vi "Generic command handler.vi"(8 "error in (no error)":errorcluster, 10 "Message in":refnum<class "GenericMessage.lvclass">, 11 "DAQMH121119OrcaFlash in":refnum<class "DAQOrcaFlash.lvclass">) -> (0 "error out":errorcluster, 2 "value":string, 3 "DAQMH121119OrcaFlash out":refnum<class "DAQOrcaFlash.lvclass">)   [LabVIEW 2012, in "DAQOrcaFlash.lvclass"]
doc: "The generic_command_handler processes the command 'generic'. Commands which are not part of the predefined list of commands fall under the 'generic' command for special activity."
uses:
  DAQOrcaFlash.lvclass
  <vilib>/Distrio/Murmex/GenericMessage/GenericMessage.lvclass
  <vilib>/Distrio/Murmex/Murmex/Murmex.lvclass
  <vilib>/Distrio/Murmex/ResetMessage/ResetMessage.lvclass
  <vilib>/Distrio/Murmex/ProceedMessage/ProceedMessage.lvclass
  DAQOrcaFlash.lvclass/DAQOrcaFlash.ctl
  <vilib>/Distrio/Murmex/Message/Message.lvclass
panel:
  # "This method is called when the GENERIC\ntrigger is sent. \n\nOverride this method when your component needs to\nrespond to this trigger. \n\nCall parent for proper implementation"
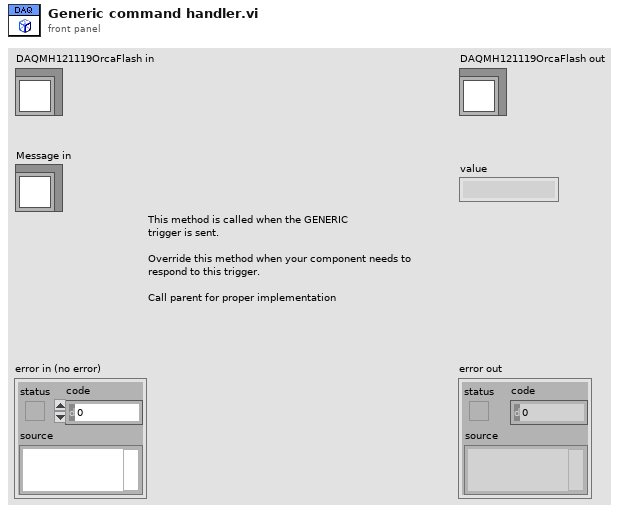
[diagram p1: front panel]
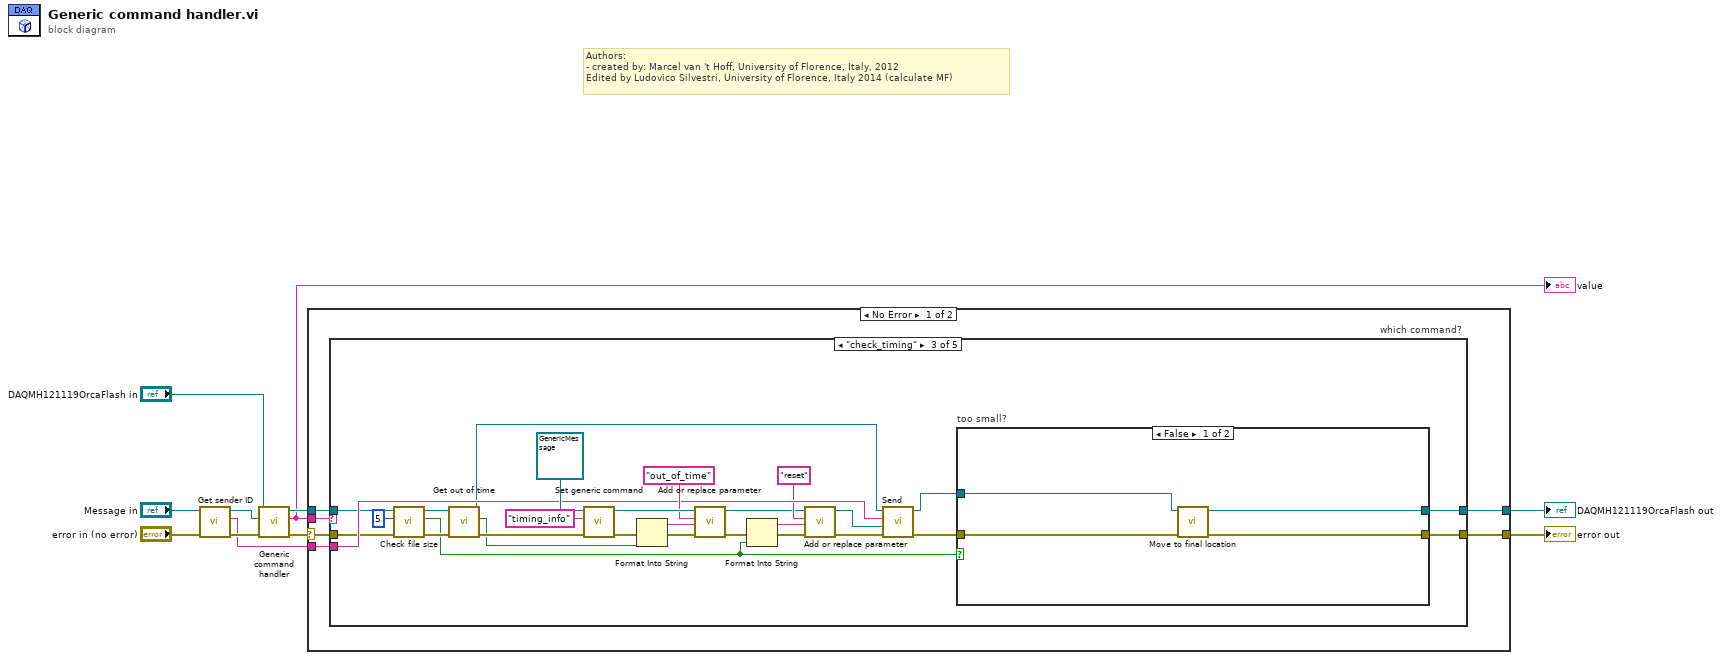
[diagram p0: block diagram]
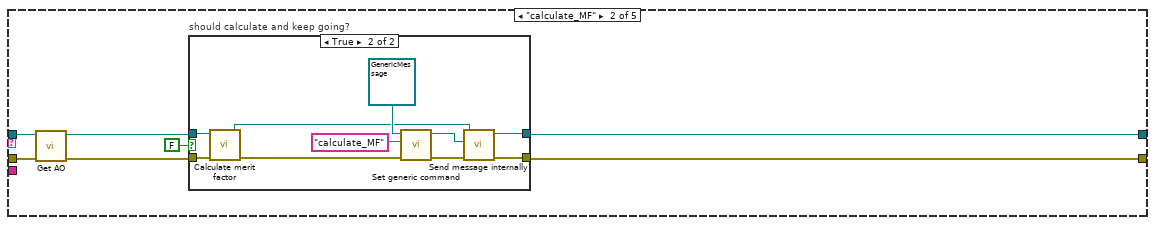
[diagram p3: hidden frame]
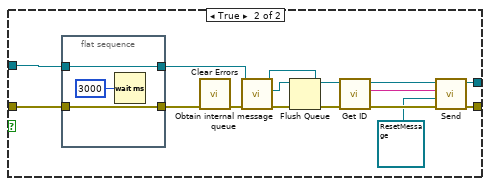
[diagram p5: hidden frame]
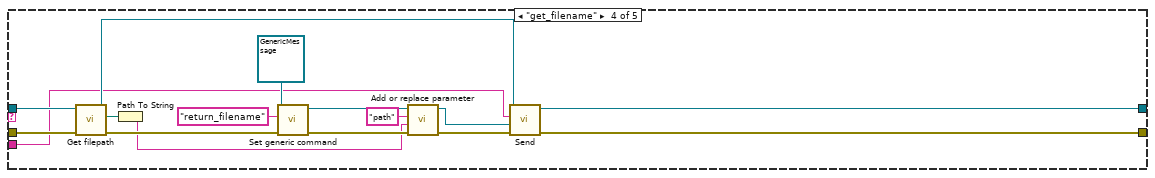
[diagram p6: hidden frame]
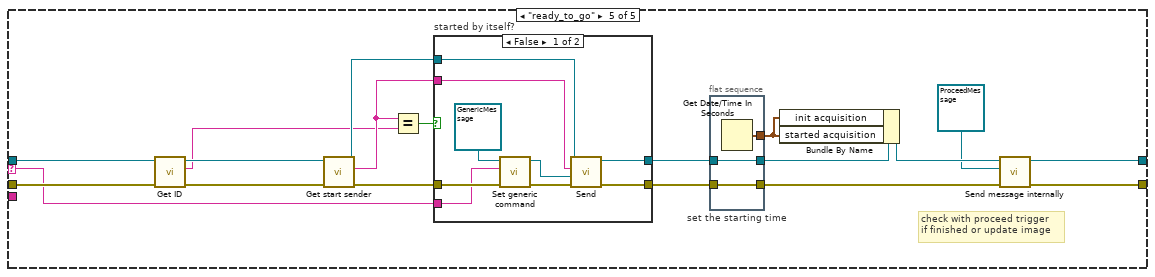
[diagram p7: hidden frame]
diagram:
  # "Authors: \n- created by: Marcel van 't Hoff, University of Florence, Italy, 2012\nEdited by Ludovico Silvestri, University of Florence, Italy 2014 (calculate MF)"
  n1 = call <vilib>:"Get sender ID.vi"("error in (no error)"="error in (no error)", "Message in"="Message in") -> ("error out"=w4:errorcluster, "sender"=w1:string, "Message out"=w2:refnum<class "GenericMessage.lvclass">)  [unwired: 7 in]
  n2 = call-parent "Generic command handler.vi"("error in (no error)"=w4, "Message in"=w2, "Murmex in"="DAQMH121119OrcaFlash in") -> ("error out"=w9:errorcluster, "value"=w5:string, "Murmex out"=w6:refnum<class "DAQOrcaFlash.lvclass">)  [unwired: 6 in]
  "value" <- w5
  n3 = case shown="No Error" w9 {
    selector: w9 -> [w16 w139]
    tunnel: [w15 w139] -> w8
    tunnel: [w14 w138] -> w7
    tunnel: w6 -> [w13 w138]
    tunnel: w5 -> [w17 _]
    tunnel: w1 -> [w12 _]
    frame No Error {
      n4 = case "which command?" shown="\"check_timing\"" w17 {
        selector: w17 -> [_ _ _ _ w121]
        tunnel: w16 -> [w19 w26 w53 w103 w123]
        tunnel: w13 -> [w18 w25 w55 w104 w118]
        tunnel: [w19 w22 w40 w89 w108] -> w15
        tunnel: [w18 w21 w41 w90 w106] -> w14
        tunnel: w12 -> [_ _ w59 w92 _]
        frame Default {
        }
        frame "calculate_MF" {
          n5 = call-dynamic "Get AO.vi"("error in (no error)"=w26, "DAQOrcaFlash in"=w25) -> ("error out"=w24:errorcluster, "DAQOrcaFlash out"=w23:refnum<class "DAQOrcaFlash.lvclass">)  [unwired: 7 in, 1 out]
          n6 = case "should calculate and keep going?" shown="True" FALSE {
            tunnel: w24 -> [w28 w38]
            tunnel: w23 -> [w27 w37]
            tunnel: [w28 w32] -> w22
            tunnel: [w27 w34] -> w21
            frame False {
            }
            frame True {
              n7 = call-dynamic "Calculate merit factor.vi"("error in (no error)"=w38, "DAQOrcaFlash in"=w37) -> ("error out"=w29:errorcluster, "DAQOrcaFlash out"=w30:refnum<class "DAQOrcaFlash.lvclass">)  [unwired: 8 in]
              n8 = call <vilib>:"Set generic command.vi"("error in (no error)"=w29, "generic command"="calculate_MF", "GenericMessage in"=refnum<class "GenericMessage.lvclass"> refnum ("GenericMessage")) -> ("error out"=w33:errorcluster, "GenericMessage out"=w31:refnum<class "GenericMessage.lvclass">)  [unwired: 7 in]
              n9 = call <vilib>:"Send message internally.vi"("error in (no error)"=w33, "Message"=w31, "Murmex in"=w30) -> ("error out"=w32:errorcluster, "Murmex out"=w34:refnum<class "DAQOrcaFlash.lvclass">)  [unwired: 7 in]
            }
          }
        }
        frame "check_timing" {
          n10 = call-dynamic "Check file size.vi"("error in (no error)"=w53, "min size (KB)"=i64 5, "DAQOrcaFlash in"=w55) -> ("error out"=w52:errorcluster, "too small?"=w39:bool, "DAQOrcaFlash out"=w54:refnum<class "DAQOrcaFlash.lvclass">)  [unwired: 6 in]
          n11 = call-dynamic "Get out of time.vi"("error in (no error)"=w52, "DAQOrcaFlash in"=w54) -> ("error out"=w58:errorcluster, "out of time?"=w56:bool, "DAQOrcaFlash out"=w57:refnum<class "DAQOrcaFlash.lvclass">)  [unwired: 7 in]
          n12 = call <vilib>:"Set generic command.vi"("error in (no error)"=w58, "generic command"="timing_info", "GenericMessage in"=refnum<class "GenericMessage.lvclass"> refnum ("Distrio Murmex 1.5:GenericMessage")) -> ("error out"=w62:errorcluster, "GenericMessage out"=w64:refnum<class "GenericMessage.lvclass">)  [unwired: 7 in]
          n13 = Format Into String(error in=w62, w56) -> (resulting string=w60:string, error out=w61:errorcluster)  [unwired: 2 in]
          n14 = call <vilib>:"Add or replace parameter.vi"("error in (no error)"=w61, "value"=w60, "name"="out_of_time", "Message in"=w64) -> ("error out"=w47:errorcluster, "Message out"=w45:refnum<class "GenericMessage.lvclass">)  [unwired: 6 in]
          n15 = Format Into String(error in=w47, w39) -> (resulting string=w48:string, error out=w49:errorcluster)  [unwired: 2 in]
          n16 = call <vilib>:"Add or replace parameter.vi"("error in (no error)"=w49, "value"=w48, "name"="reset", "Message in"=w45) -> ("error out"=w46:errorcluster, "Message out"=w44:refnum<class "GenericMessage.lvclass">)  [unwired: 6 in]
          n17 = call <vilib>:"Send.vi"("error in (no error)"=w46, "Message"=w44, "recipient"=w59, "Murmex in"=w57) -> ("error out"=w42:errorcluster, "Murmex out"=w43:refnum<class "DAQOrcaFlash.lvclass">)  [unwired: 6 in]
          n18 = case "too small?" shown="False" w39 {
            tunnel: w42 -> [w70 w81]
            tunnel: w43 -> [w68 w79]
            tunnel: [w69 w77] -> w40
            tunnel: [w67 w73] -> w41
            frame False {
              n19 = call-dynamic "Move to final location.vi"("error in (no error)"=w70, "DAQOrcaFlash in"=w68) -> ("error out"=w69:errorcluster, "DAQOrcaFlash out"=w67:refnum<class "DAQOrcaFlash.lvclass">)  [unwired: 8 in]
            }
            frame True {
              n20 = flat-sequence {
                tunnel: [w88] -> w82
                tunnel: w81 -> [w88]
                tunnel: [w87] -> w80
                tunnel: w79 -> [w87]
                frame #0 {
                  n21 = Wait (ms)(milliseconds to wait=u32 3000) -> ()  [unwired: 1 out]
                }
              }
              n22 = call <vilib>:"Clear Errors.vi"("error in (no error)"=w82) -> ("error out"=w85:errorcluster)  [unwired: 6 in]
              n23 = call <vilib>:"Obtain internal message queue.vi"("error in (no error)"=w85, "Murmex in"=w80) -> ("error out"=w83:errorcluster, "internal message queue"=w84:refnum<queue>, "Murmex out"=w75:refnum<class "DAQOrcaFlash.lvclass">)  [unwired: 7 in]
              n24 = Flush Queue(queue=w84, error in (no error)=w83) -> (error out=w76:errorcluster)  [unwired: 2 out]
              n25 = call <vilib>:"Get ID.vi"("error in (no error)"=w76, "Murmex in"=w75) -> ("error out"=w78:errorcluster, "component id"=w72:string, "Murmex out"=w74:refnum<class "DAQOrcaFlash.lvclass">)  [unwired: 7 in]
              n26 = call <vilib>:"Send.vi"("error in (no error)"=w78, "Message"=refnum<class "ResetMessage.lvclass"> refnum ("Message in"), "recipient"=w72, "Murmex in"=w74) -> ("error out"=w77:errorcluster, "Murmex out"=w73:refnum<class "DAQOrcaFlash.lvclass">)  [unwired: 6 in]
            }
          }
        }
        frame "get_filename" {
          n27 = call "Get filepath.vi"("error in (no error)"=w103, "DAQOrcaFlash in"=w104) -> ("error out"=w100:errorcluster, "full storage path"=w96:path, "DAQOrcaFlash out"=w93:refnum<class "DAQOrcaFlash.lvclass">)  [unwired: 7 in]
          n28 = Path To String(path=w96) -> (string=w95:string)
          n29 = call <vilib>:"Set generic command.vi"("error in (no error)"=w100, "generic command"="return_filename", "GenericMessage in"=refnum<class "GenericMessage.lvclass"> refnum ("Message in")) -> ("error out"=w99:errorcluster, "GenericMessage out"=w98:refnum<class "GenericMessage.lvclass">)  [unwired: 7 in]
          n30 = call <vilib>:"Add or replace parameter.vi"("error in (no error)"=w99, "value"=w95, "name"="path", "Message in"=w98) -> ("error out"=w94:errorcluster, "Message out"=w91:refnum<class "GenericMessage.lvclass">)  [unwired: 6 in]
          n31 = call <vilib>:"Send.vi"("error in (no error)"=w94, "Message"=w91, "recipient"=w92, "Murmex in"=w93) -> ("error out"=w89:errorcluster, "Murmex out"=w90:refnum<class "DAQOrcaFlash.lvclass">)  [unwired: 6 in]
        }
        frame "ready_to_go" {
          # "check with proceed trigger\nif finished or update image"
          n32 = call <vilib>:"Get ID.vi"("error in (no error)"=w123, "Murmex in"=w118) -> ("error out"=w119:errorcluster, "component id"=w114:string, "Murmex out"=w117:refnum<class "DAQOrcaFlash.lvclass">)  [unwired: 7 in]
          n33 = call-dynamic "Get start sender.vi"("error in (no error)"=w119, "DAQOrcaFlash in"=w117) -> ("error out"=w122:errorcluster, "start sender"=w115:string, "DAQOrcaFlash out"=w120:refnum<class "DAQOrcaFlash.lvclass">)  [unwired: 7 in]
          n34 = Equal?(x=w115, y=w114) -> (x = y?=w116:bool)
          n35 = case "started by itself?" shown="False" w116 {
            tunnel: w122 -> [w132 w136]
            tunnel: w121 -> [w131 _]
            tunnel: w120 -> [w130 w137]
            tunnel: w115 -> [w129 _]
            tunnel: [w128 w137] -> w109
            tunnel: [w127 w136] -> w111
            frame False {
              n36 = call <vilib>:"Set generic command.vi"("error in (no error)"=w132, "generic command"=w131, "GenericMessage in"=refnum<class "GenericMessage.lvclass"> refnum ("Distrio Murmex 1.2:GenericMessage")) -> ("error out"=w135:errorcluster, "GenericMessage out"=w133:refnum<class "GenericMessage.lvclass">)  [unwired: 7 in]
              n37 = call <vilib>:"Send.vi"("error in (no error)"=w135, "Message"=w133, "recipient"=w129, "Murmex in"=w130) -> ("error out"=w127:errorcluster, "Murmex out"=w128:refnum<class "DAQOrcaFlash.lvclass">)  [unwired: 6 in]
            }
            frame True {
            }
          }
          n38 = flat-sequence "set the starting time" {
            tunnel: [w126] -> w113
            tunnel: w109 -> [w126]
            tunnel: w111 -> [w125]
            tunnel: [w125] -> w110
            tunnel: [w124] -> w112
            frame #0 {
              n39 = Get Date/Time In Seconds() -> (seconds since 1Jan1904=w124:timestamp)
            }
          }
          n40 = Bundle By Name(cluster=w113, "init acquisition"=w112, "started acquisition"=w112) -> (w107:refnum<class "DAQOrcaFlash.lvclass">)
          n41 = call <vilib>:"Send message internally.vi"("error in (no error)"=w110, "Message"=refnum<class "ProceedMessage.lvclass"> refnum ("ProceedMessage"), "Murmex in"=w107) -> ("error out"=w108:errorcluster, "Murmex out"=w106:refnum<class "DAQOrcaFlash.lvclass">)  [unwired: 7 in]
        }
      }
    }
    frame Error {
    }
  }
  "error out" <- w8
  "DAQMH121119OrcaFlash out" <- w7
